vi "getRef.vi"(8 "error in":errorcluster, 10 "name":string, 11 "Gen ref in":refnum<vi>) -> (0 "error out":errorcluster, 2 "cousins":string, 3 "Gen ref out":refnum<vi>)   [LabVIEW 2017]
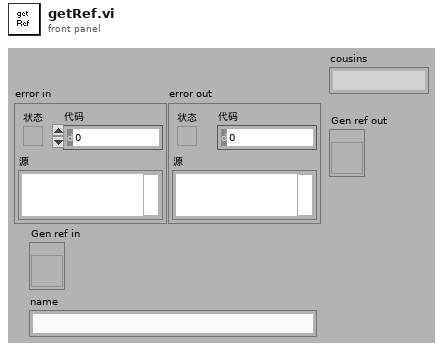
[diagram p1: front panel]
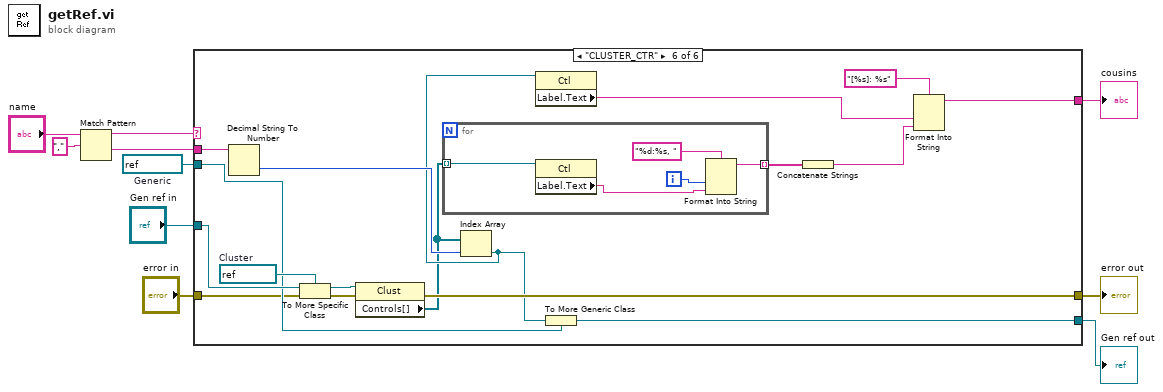
[diagram p0: block diagram]
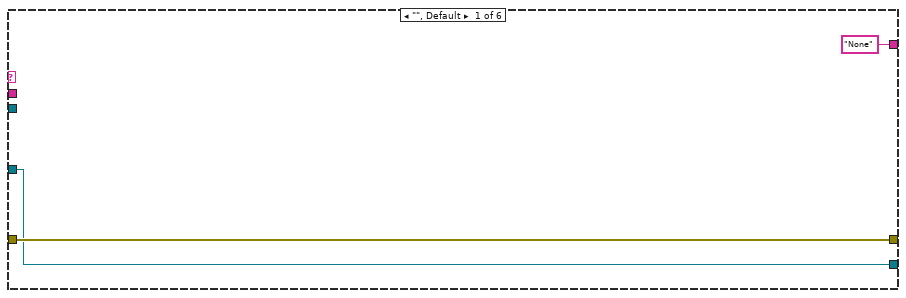
[diagram p2: hidden frame]
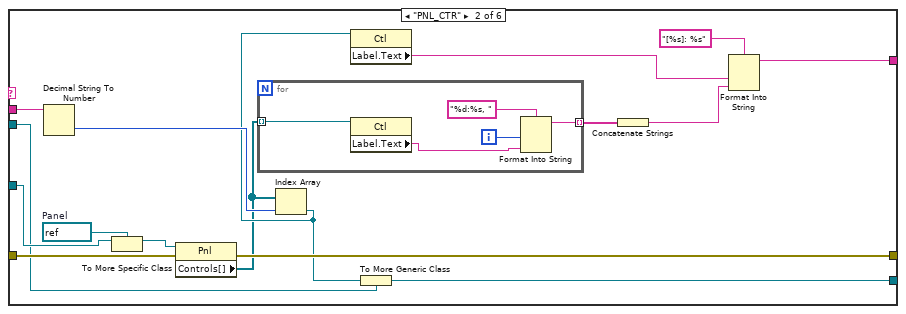
[diagram p3: hidden frame]
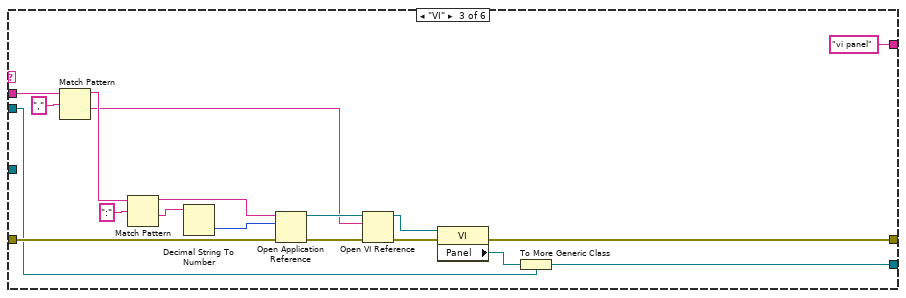
[diagram p4: hidden frame]
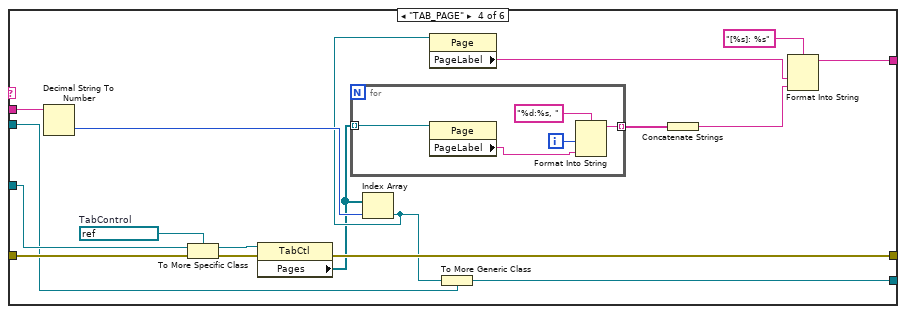
[diagram p5: hidden frame]
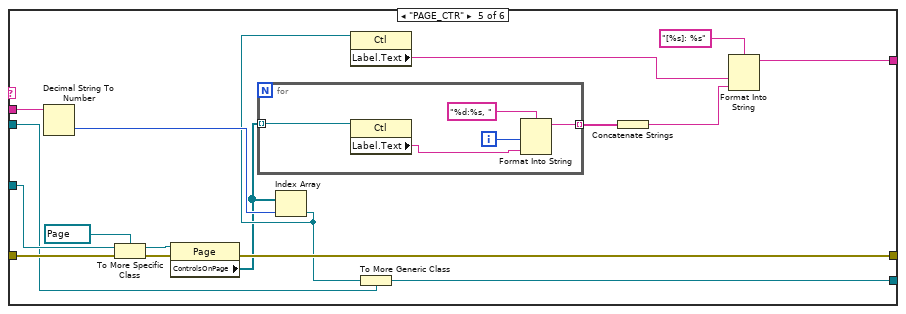
[diagram p6: hidden frame]
diagram:
  w3 = refnum<vi> refnum  # Generic
  n1 = Match Pattern(string="name", regular expression="," ("正则表达式")) -> (before substring=w6:string, after substring=w5:string)  [unwired: 3 out]
  n2 = case shown="\"CLUSTER_CTR\"" w6 {
    tunnel: "error in" -> [w13 w25 w48 w66 w85 w106]
    tunnel: [w13 w22 w37 w62 w83 w105] -> w9
    tunnel: w5 -> [_ w24 w47 w65 w87 w107]
    tunnel: [w12 w29 w40 w64 w88 w104] -> w2
    tunnel: "Gen ref in" -> [w12 w28 _ w67 w90 w110]
    tunnel: w3 -> [_ w21 w36 w61 w82 w108]
    tunnel: ["None" ("Label.Text") w14 "vi panel" ("Label.Text") w54 w75 w97] -> w1
    frame "", Default {
    }
    frame "PNL_CTR" {
      w27 = refnum<vi> refnum  # Panel
      n3 = Decimal String To Number(string=w24) -> (number=w23:i32)  [unwired: 3 out]
      n4 = To More Specific Class(target class=w27, reference=w28) -> (specific class reference=w26:refnum<vi>)  [unwired: 1 in, 1 out]
      n5 = property class="Pnl"(reference=w26, error in=w25) -> (error out=w22:errorcluster, "Controls[]"=w19:refnum<vi>[])  [unwired: 1 out]
      n6 = for {
        tunnel: w19 -> [w34] mode=indexing
        tunnel: [w30] -> w16 mode=indexing
        i -> [w32]
        n7 = property class="Ctl"(reference=w34) -> ("Label.Text"=w31:string)  [unwired: 1 in, 2 out]
        n8 = Format Into String(format string="%d:%s, ", w32, w31) -> (resulting string=w30:string)  [unwired: 2 in, 1 out]
      }
      n9 = Index Array(array=w19, index=w23) -> (element=w20:refnum<vi>)
      n10 = property class="Ctl"(reference=w20) -> ("Label.Text"=w15:string)  [unwired: 1 in, 2 out]
      n11 = To More Generic Class(target class=w21, reference=w20) -> (generic class reference=w29:refnum<vi>)
      n12 = Concatenate Strings(w16) -> (w18:string)
      n13 = Format Into String(format string="[%s]: %s", w15, w18) -> (resulting string=w14:string)  [unwired: 2 in, 1 out]
    }
    frame "VI" {
      n14 = Match Pattern(string=w47, regular expression="," ("正则表达式")) -> (before substring=w44:string, after substring=w42:string)  [unwired: 3 out]
      n15 = Match Pattern(string=w44, regular expression=":" ("正则表达式")) -> (before substring=w43:string, after substring=w39:string)  [unwired: 3 out]
      n16 = Decimal String To Number(string=w39) -> (number=w38:i32)  [unwired: 3 out]
      n17 = Open Application Reference(8:w48, 10:w38, 11:w43) -> (0:w50:errorcluster, 3:w51:refnum<vi>)  [unwired: 1 out]
      n18 = Open VI Reference(application reference (local)=w51, vi path=w42, error in (no error)=w50) -> (vi reference=w52:refnum<vi>, error out=w49:errorcluster)  [unwired: 3 out]
      n19 = property class="VI"(reference=w52, error in=w49) -> (error out=w37:errorcluster, "Panel"=w41:refnum<vi>)  [unwired: 1 out]
      n20 = To More Generic Class(target class=w36, reference=w41) -> (generic class reference=w40:refnum<vi>)
    }
    frame "TAB_PAGE" {
      w68 = refnum<vi> refnum  # TabControl
      n21 = Decimal String To Number(string=w65) -> (number=w63:i32)  [unwired: 3 out]
      n22 = To More Specific Class(target class=w68, reference=w67, error in=w66) -> (specific class reference=w59:refnum<vi>, error out=w69:errorcluster)
      n23 = property class="TabCtl"(reference=w59, error in=w69) -> (error out=w62:errorcluster, "Pages"=w58:refnum<vi>[])  [unwired: 1 out]
      n24 = for {
        tunnel: w58 -> [w74] mode=indexing
        tunnel: [w71] -> w57 mode=indexing
        i -> [w72]
        n25 = property class="Page"(reference=w74) -> ("PageLabel"=w73:string)  [unwired: 1 in, 2 out]
        n26 = Format Into String(format string="%d:%s, ", w72, w73) -> (resulting string=w71:string)  [unwired: 2 in, 1 out]
      }
      n27 = Index Array(array=w58, index=w63) -> (element=w60:refnum<vi>)
      n28 = property class="Page"(reference=w60) -> ("PageLabel"=w56:string)  [unwired: 1 in, 2 out]
      n29 = To More Generic Class(target class=w61, reference=w60) -> (generic class reference=w64:refnum<vi>)
      n30 = Concatenate Strings(w57) -> (w55:string)
      n31 = Format Into String(format string="[%s]: %s", w56, w55) -> (resulting string=w54:string)  [unwired: 2 in, 1 out]
    }
    frame "PAGE_CTR" {
      n32 = Decimal String To Number(string=w87) -> (number=w86:i32)  [unwired: 3 out]
      n33 = To More Specific Class(target class=refnum<vi> refnum ("元素"), reference=w90, error in=w85) -> (specific class reference=w89:refnum<vi>, error out=w91:errorcluster)
      n34 = property class="Page"(reference=w89, error in=w91) -> (error out=w83:errorcluster, "ControlsOnPage"=w80:refnum<vi>[])  [unwired: 1 out]
      n35 = for {
        tunnel: w80 -> [w96] mode=indexing
        tunnel: [w92] -> w79 mode=indexing
        i -> [w93]
        n36 = property class="Ctl"(reference=w96) -> ("Label.Text"=w94:string)  [unwired: 1 in, 2 out]
        n37 = Format Into String(format string="%d:%s, ", w93, w94) -> (resulting string=w92:string)  [unwired: 2 in, 1 out]
      }
      n38 = Index Array(array=w80, index=w86) -> (element=w81:refnum<vi>)
      n39 = property class="Ctl"(reference=w81) -> ("Label.Text"=w76:string)  [unwired: 1 in, 2 out]
      n40 = To More Generic Class(target class=w82, reference=w81) -> (generic class reference=w88:refnum<vi>)
      n41 = Concatenate Strings(w79) -> (w77:string)
      n42 = Format Into String(format string="[%s]: %s", w76, w77) -> (resulting string=w75:string)  [unwired: 2 in, 1 out]
    }
    frame "CLUSTER_CTR" {
      w109 = refnum<vi> refnum  # Cluster
      n43 = Decimal String To Number(string=w107) -> (number=w111:i32)  [unwired: 3 out]
      n44 = To More Specific Class(target class=w109, reference=w110, error in=w106) -> (specific class reference=w112:refnum<vi>, error out=w113:errorcluster)
      n45 = property class="Clust"(reference=w112, error in=w113) -> (error out=w105:errorcluster, "Controls[]"=w99:refnum<vi>[])  [unwired: 1 out]
      n46 = for {
        tunnel: w99 -> [w118] mode=indexing
        tunnel: [w114] -> w102 mode=indexing
        i -> [w115]
        n47 = property class="Ctl"(reference=w118) -> ("Label.Text"=w116:string)  [unwired: 1 in, 2 out]
        n48 = Format Into String(format string="%d:%s, ", w115, w116) -> (resulting string=w114:string)  [unwired: 2 in, 1 out]
      }
      n49 = Index Array(array=w99, index=w111) -> (element=w103:refnum<vi>)
      n50 = property class="Ctl"(reference=w103) -> ("Label.Text"=w98:string)  [unwired: 1 in, 2 out]
      n51 = To More Generic Class(target class=w108, reference=w103) -> (generic class reference=w104:refnum<vi>)
      n52 = Concatenate Strings(w102) -> (w100:string)
      n53 = Format Into String(format string="[%s]: %s", w98, w100) -> (resulting string=w97:string)  [unwired: 2 in, 1 out]
    }
  }
  "error out" <- w9
  "Gen ref out" <- w2
  "cousins" <- w1
